vi "GENser Meas Output Voltage.vi"(7 "GEN Addr":i16=-1, 8 "error":errorcluster, 11 "VISA":refnum<visa-resource-name>) -> (0 "error out":errorcluster, 2 "Output Voltage":dbl format="%.4f", 3 "VISA out":refnum<visa-resource-name>)   [LabVIEW 2017]
doc: "This VI returns the output voltage measured by the power supply. \n(query \"MV?\")"
panel:
  # "Lambda Genesys \nSerial Port\n  DC Power Supplies"
  # "Measure the \nOutput Voltage"
  # "-1 = no address change"
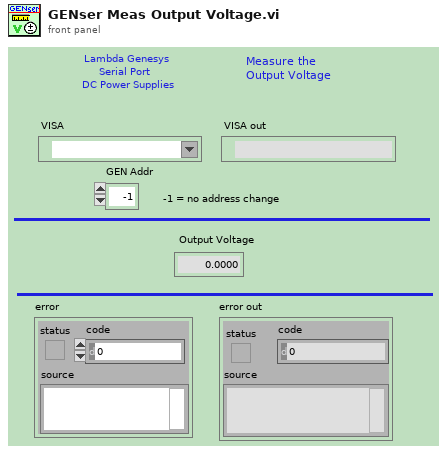
[diagram p1: front panel]
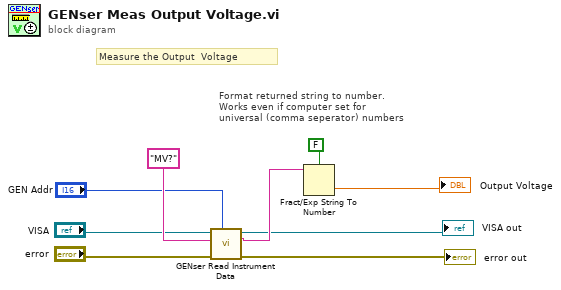
[diagram p0: block diagram]
diagram:
  # "Format returned string to number.\nWorks even if computer set for \nuniversal (comma seperator) numbers"
  # "Measure the Output  Voltage"
  n1 = call "GENser Read Instrument Data.vi"("GEN Addr"="GEN Addr", "error"="error", "Query"="MV?" ("format string"), "VISA"="VISA") -> ("error out"=→"error out":errorcluster, "Response"=w7:string, "VISA out"=→"VISA out":refnum<visa-resource-name>)  [unwired: 4 in, 1 out]
  n2 = Fract/Exp String To Number(use system decimal point (T)=FALSE, string=w7) -> (number=→"Output Voltage":dbl)  [unwired: 2 in, 1 out]
